vi "Poisson PF.vi"(10 "lambda":dbl=1.0, 11 "x":i32=1) -> (0 "error":i32, 3 "prob(x)":dbl=0.36787944117144233)   [LabVIEW 2020, in "NI_Gmath.lvlib"]
doc: "Computes the discrete probability function (PF), or the probability that the random variate X, where X describes the selected distribution type, takes on the value <B>n</B>. You must manually select the polymorphic instance to use."
uses:
  <vilib>/gmath/NI_Gmath.lvlib
panel:
  # "Poisson PF"
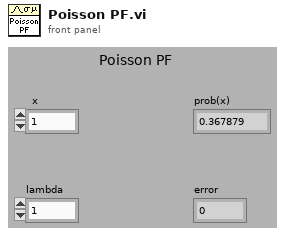
[diagram p1: front panel]
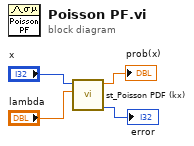
[diagram p0: block diagram]
diagram:
  n1 = call <vilib>:"st_Poisson PDF (kx).vi"("a"="lambda", "x"="x") -> ("error"=→"error":i32, "pdf(x)"=→"prob(x)":dbl)  [unwired: 8 in]
